vi "Open device.vi"(2 "error in (no error)":errorcluster, 3 "location":u32, 4 "channel":string, 5 "name":string) -> (0 "error out":errorcluster, 1 "handle":u32)   [LabVIEW 2013]
uses:
  lib/FTCSPI.dll
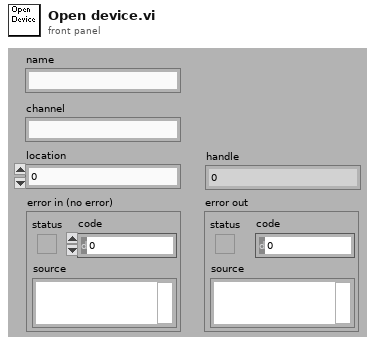
[diagram p1: front panel]
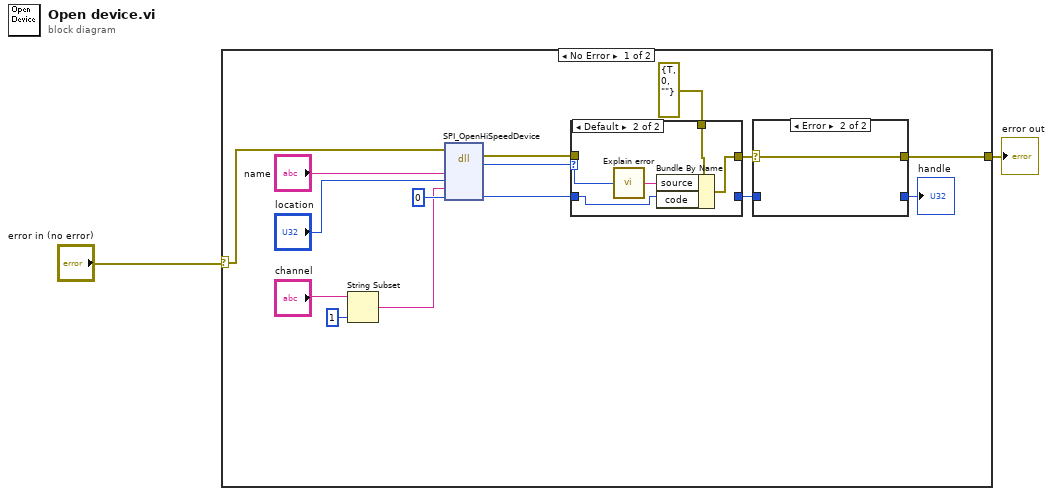
[diagram p0: block diagram]
diagram:
  n1 = case shown="No Error" "error in (no error)" {
    selector: "error in (no error)" -> [w15 w28]
    tunnel: [w8 w28] -> w1
    frame No Error {
      n2 = String Subset(string="channel", length (rest)=1 ("length (rest)")) -> (substring=w4:string)  [unwired: 1 out]
      n3 = dll-call lib="C:/Users/SuperUser/Documents/HiSparc/hisparcdaq/FPGA/lib/FTCSPI.dll" fn="SPI_OpenHiSpeedDevice"(error in=w15, "name"="name", "location"="location", "channel"=w4, "handle"=u32 0) -> (error out=w12:errorcluster, "result"=w14:u32, "handle"=w13:u32)  [unwired: 4 in, 2 out]
      n4 = case shown="Default" w14 {
        selector: w14 -> [_ w27]
        tunnel: w13 -> [w22 w23]
        tunnel: w12 -> [w21 _]
        tunnel: [w22 _] -> w9
        tunnel: [w21 w24] -> w10
        tunnel: errorcluster {"status"=TRUE, "code"=0, "source"=""} ("error out") -> [_ w26]
        frame 0 {
        }
        frame Default {
          n5 = call "Explain error.vi"("error"=w27) -> ("error string"=w25:string)
          n6 = Bundle By Name(cluster=w26, "source"=w25, "code"=w23) -> (w24:errorcluster)
        }
      }
      n7 = case shown="Error" w10 {
        selector: w10 -> [w19 w20]
        tunnel: [w19 w20] -> w8
        tunnel: w9 -> [w18 _]
        tunnel: [w18 _] -> w7
        frame No Error {
        }
        frame Error {
        }
      }
      "handle" <- w7
    }
    frame Error {
    }
  }
  "error out" <- w1
